vi "Linux Native Sleep Performance Test.vi"() -> ()   [LabVIEW 2021]
uses:
  <vilib>/Platform/TimedLoop/XDataNode/timing_clust.ctl
  <vilib>/Platform/TimedLoop/XDataNode/nitl_modes.ctl
  <vilib>/Platform/TimedLoop/XDataNode/wakeup.ctl
  <vilib>/NI/NI Linux RT Utilities/Controls/Public/nanosleep flags.ctl
  <vilib>/NI/NI Linux RT Utilities/Controls/Public/C Enums/clockid_t.ctl
  <vilib>/NI/NI Linux RT Utilities/VIs/Private/C Functions/clock_nanosleep.vi
  <vilib>/NI/NI Linux RT Utilities/VIs/Public/Convert Types/convert nanoseconds to timespec.vi
  <vilib>/NI/NI Linux RT Errno/VIs/Public/Generate LabVIEW Error from Errno.vi
  <vilib>/NI/NI Linux RT Errno/VIs/Public/Get Errno Value for Calling Thread.vi
  <vilib>/NI/NI Linux RT Errno/VIs/Public/Get LV Error Info from Errno.vi
  <vilib>/Utility/error.llb/Error Cluster From Error Code.vi
  <vilib>/Platform/TimedLoop/XDataNode/XDataNode.xnode
  <vilib>/Platform/TimedLoop/XDataNode/XDNodeRunTimeDep.lvlib
  <vilib>/NI/NI Linux RT Utilities/Linux RT Utilities.lvlib
panel:
  out "avg Linux Sleep":dbl
  out "max Linux Sleep":dbl
  out "avg RT Sleep":dbl
  out "max RT Sleep":dbl
  out "pass":bool
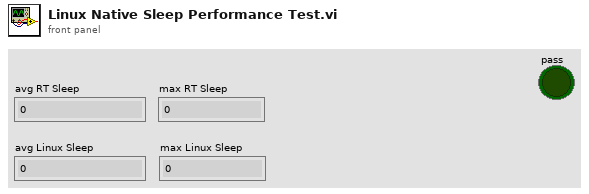
[diagram p1: front panel]
types:
  T1 = typedef "XDNodeRunTimeDep.lvlib/timing_clust.ctl" = cluster{"Expected End [f-1]":u64, "Actual End [f-1]":u64, "Finished Late? [f-1]":bool, "Expected End [i-1]":u64, "Actual End [i-1]":u64, "Finished Late? [i-1]":bool, "Expected Start [i]":u64, "Actual Start [i]":u64, "Expected Start [f]":u64, "Actual Start [f]":u64, "Source Name":string, "Structure Name":string, "Period":i64, "Deadline":i64, "Offset":i64, "Start":i64, "Priority":i32, "Timeout":i32, "Mode":T2, "Wakeup Reason":T3, "Error":errorcluster, "Source Type":string, "Secondary Source Type":string, "Global End Time":u64, "Global Start Time":u64, "Frame Duration":u64, "Iteration Duration":u64, "Assigned CPU":i32, "I/O Scan Engine Mode":u32}
  T2 = typedef "XDNodeRunTimeDep.lvlib/nitl_modes.ctl" = enum32{"No Change", "Process missed periods, maintain original phase", "Discard missed periods, maintain original phase", "Process missed periods, ignore original phase", "Discard missed periods, ignore original phase"}
  T3 = typedef "XDNodeRunTimeDep.lvlib/wakeup.ctl" = enum32{"Normal", "Aborted", "Asynchronous wakeup", "Timing source error", "Timed loop error", "Timeout"}
  T4 = typedef "Linux RT Utilities.lvlib/clockid_t.ctl" = enum16{"Realtime", "Monotonic"}
  T5 = typedef "Linux RT Utilities.lvlib/nanosleep flags.ctl" = enum16{"Relative Time", "Absolute Time"}
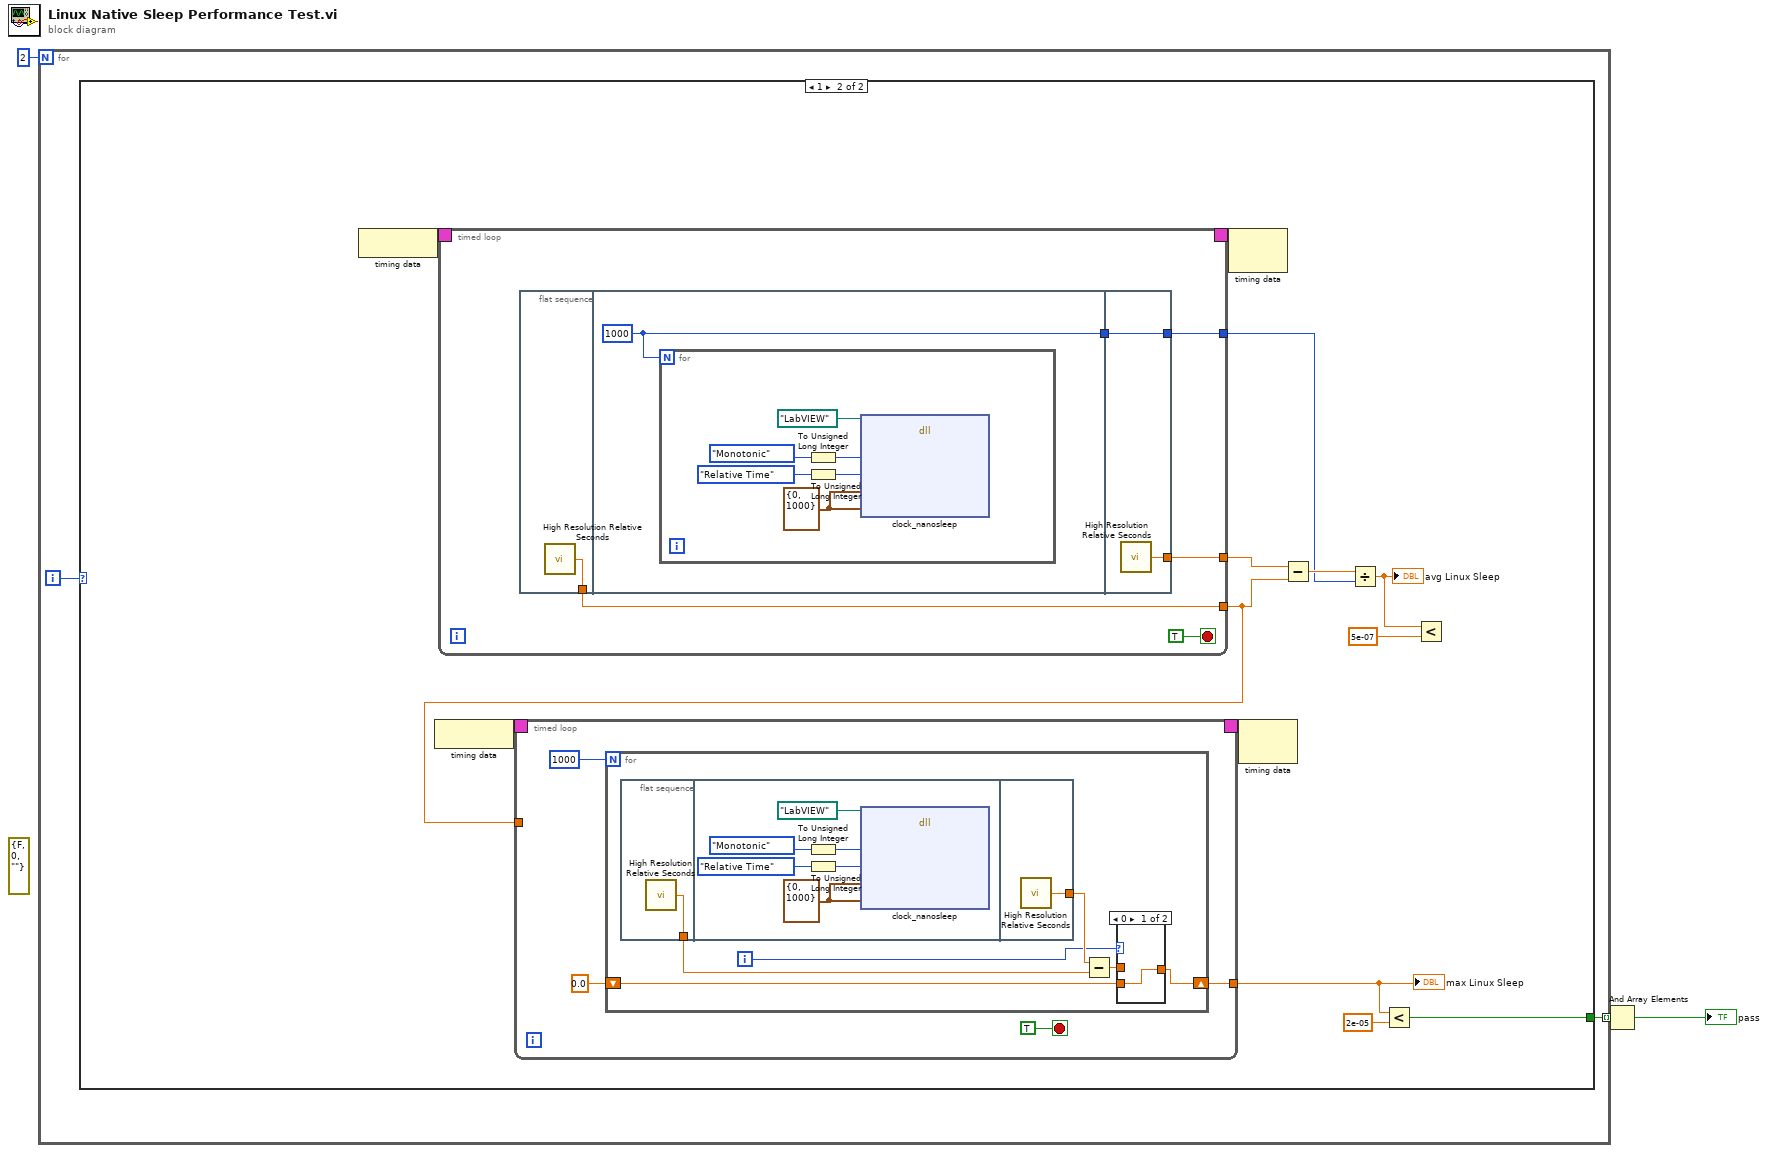
[diagram p0: block diagram]
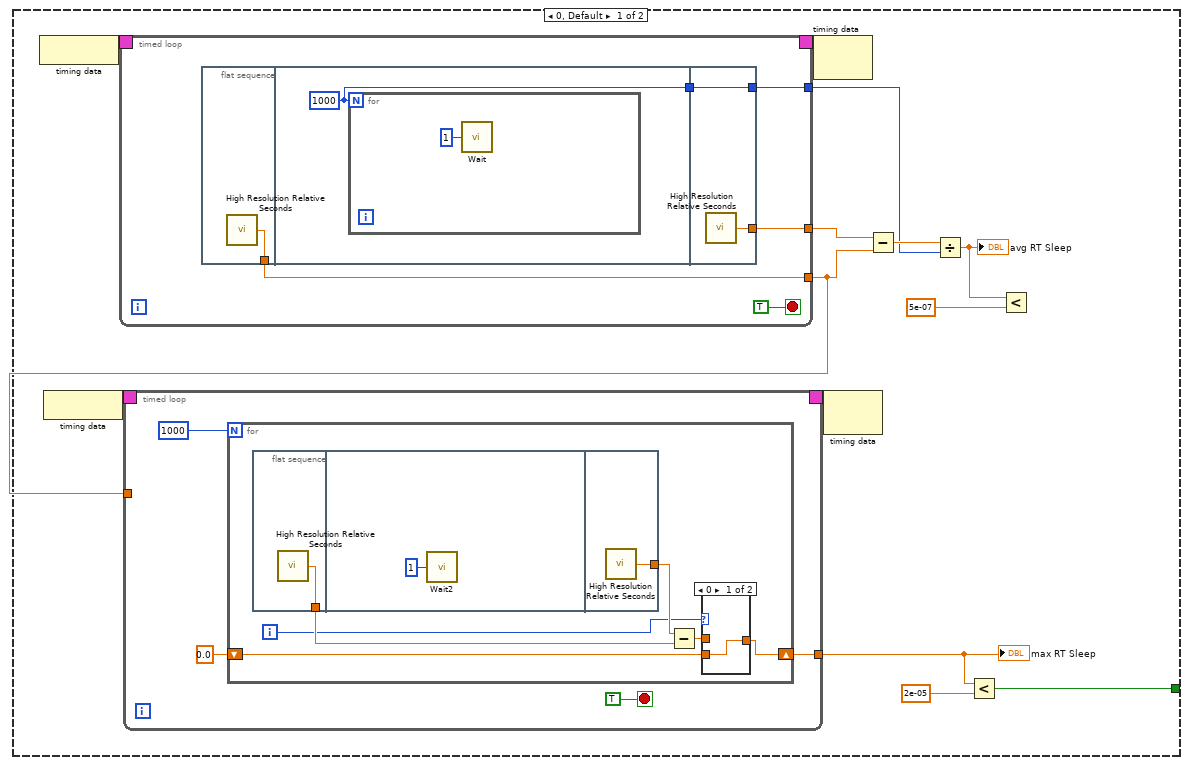
[diagram p2: hidden frame]
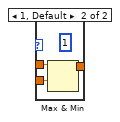
[diagram p3: hidden frame]
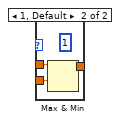
[diagram p4: hidden frame]
diagram:
  (unwired) errorcluster {"status"=FALSE, "code"=0, "source"=""} ("error out")
  n1 = for {
    N: 2 -> [_]
    tunnel: [w5] -> w2 mode=indexing
    i -> [w4]
    n2 = case shown="1" w4 {
      tunnel: [w7 w55] -> w5
      frame 0, Default {
        n3 = node-c288() -> (w18:T1)
        n4 = node-c288() -> (w16:T1)
        n5 = timed-loop {
          timing: w18 -> [_]
          timing-out: [_] -> w17
          tunnel: [w43] -> w14
          tunnel: [w42] -> w6
          tunnel: [w41] -> w12
          stop <- TRUE stop-if-true
          n6 = flat-sequence {
            tunnel: [w45] -> w42
            tunnel: [w46] -> w40
            tunnel: [w49] -> w43
            tunnel: [w48] -> w41
            tunnel: w40 -> [w48]
            frame #0 {
              n7 = call <vilib>:"High Resolution Relative Seconds.vi"() -> ("relative seconds"=w45:dbl)
            }
            frame #1 {
              w46 = 1000
              n8 = for {
                N: w46 -> [_]
                n9 = call "Wait"("Count(uSec)"=u32 1) -> ()  [unwired: 1 out]
              }
            }
            frame #2 {
              n10 = call <vilib>:"High Resolution Relative Seconds.vi"() -> ("relative seconds"=w49:dbl)
            }
          }
        }
        n11 = timed-loop {
          timing: w16 -> [_]
          timing-out: [_] -> w15
          tunnel: [w19] -> w9
          tunnel: w6 -> [_]
          stop <- TRUE stop-if-true
          n12 = for {
            N: 1000 -> [_]
            shift-right: [w24] -> w19
            shift-left: 0.0 -> [w25]
            i -> [w23]
            n13 = flat-sequence {
              tunnel: [w33] -> w27
              tunnel: [w35] -> w28
              frame #0 {
                n14 = call <vilib>:"High Resolution Relative Seconds.vi"() -> ("relative seconds"=w33:dbl)
              }
              frame #1 {
                n15 = call "Wait2"("Count(uSec)"=u32 1) -> ()  [unwired: 1 out]
              }
              frame #2 {
                n16 = call <vilib>:"High Resolution Relative Seconds.vi"() -> ("relative seconds"=w35:dbl)
              }
            }
            n17 = Subtract(x=w28, y=w27) -> (x-y=w26:dbl)
            n18 = case shown="0" w23 {
              tunnel: w26 -> [_ w32]
              tunnel: w25 -> [w29 w31]
              tunnel: [w29 w30] -> w24
              frame 0 {
              }
              frame 1, Default {
                (unwired) u32 1 ("milliseconds to wait")
                n19 = Max & Min(x=w32, y=w31) -> (max(x,y)=w30:dbl)  [unwired: 1 out]
              }
            }
          }
        }
        "max RT Sleep" <- w9
        n20 = node-c288(w17) -> ()  [unwired: 1 out]
        n21 = node-c288(w15) -> ()  [unwired: 1 out]
        n22 = Subtract(x=w14, y=w6) -> (x-y=w13:dbl)
        n23 = Divide(x=w13, y=w12) -> (x/y=w11:dbl)
        "avg RT Sleep" <- w11
        n24 = Less?(x=w9, y=2e-05) -> (x < y?=w7:bool)
        n25 = Less?(x=w11, y=5e-07) -> ()  [unwired: 1 out]
      }
      frame 1 {
        n26 = node-c288() -> (w66:T1)
        n27 = node-c288() -> (w64:T1)
        n28 = timed-loop {
          timing: w66 -> [_]
          timing-out: [_] -> w65
          tunnel: [w96] -> w62
          tunnel: [w95] -> w54
          tunnel: [w94] -> w60
          stop <- TRUE stop-if-true
          n29 = flat-sequence {
            tunnel: [w98] -> w95
            tunnel: [w99] -> w93
            tunnel: [w107] -> w96
            tunnel: [w106] -> w94
            tunnel: w93 -> [w106]
            frame #0 {
              n30 = call <vilib>:"High Resolution Relative Seconds.vi"() -> ("relative seconds"=w98:dbl)
            }
            frame #1 {
              w99 = 1000
              n31 = for {
                N: w99 -> [_]
                w100 = cluster{"sec":i64, "nsec":i64} {"sec"=0, "nsec"=1000} ("request")
                n32 = To Unsigned Long Integer(number=clockid_t."Monotonic" ("clockid_t")) -> (unsigned 32bit integer=w102:u32)
                n33 = To Unsigned Long Integer(number=nanosleep_flags."Relative Time" ("flags")) -> (unsigned 32bit integer=w101:u32)
                n34 = dll-call lib="?" fn="clock_nanosleep"(path in=path "LabVIEW" ("Path"), "clockid_t"=w102, "flags"=w101, "request"=w100, "remain"=w100) -> ()  [unwired: 7 in, 2 out]
              }
            }
            frame #2 {
              n35 = call <vilib>:"High Resolution Relative Seconds.vi"() -> ("relative seconds"=w107:dbl)
            }
          }
        }
        n36 = timed-loop {
          timing: w64 -> [_]
          timing-out: [_] -> w63
          tunnel: [w67] -> w57
          tunnel: w54 -> [_]
          stop <- TRUE stop-if-true
          n37 = for {
            N: 1000 -> [_]
            shift-right: [w72] -> w67
            shift-left: 0.0 -> [w73]
            i -> [w71]
            n38 = flat-sequence {
              tunnel: [w81] -> w75
              tunnel: [w88] -> w76
              frame #0 {
                n39 = call <vilib>:"High Resolution Relative Seconds.vi"() -> ("relative seconds"=w81:dbl)
              }
              frame #1 {
                w87 = cluster{"sec":i64, "nsec":i64} {"sec"=0, "nsec"=1000} ("request")
                n40 = To Unsigned Long Integer(number=clockid_t."Monotonic" ("clockid_t")) -> (unsigned 32bit integer=w85:u32)
                n41 = To Unsigned Long Integer(number=nanosleep_flags."Relative Time" ("flags")) -> (unsigned 32bit integer=w86:u32)
                n42 = dll-call lib="?" fn="clock_nanosleep"(path in=path "LabVIEW" ("Path"), "clockid_t"=w85, "flags"=w86, "request"=w87, "remain"=w87) -> ()  [unwired: 7 in, 2 out]
              }
              frame #2 {
                n43 = call <vilib>:"High Resolution Relative Seconds.vi"() -> ("relative seconds"=w88:dbl)
              }
            }
            n44 = Subtract(x=w76, y=w75) -> (x-y=w74:dbl)
            n45 = case shown="0" w71 {
              tunnel: w74 -> [_ w80]
              tunnel: w73 -> [w77 w79]
              tunnel: [w77 w78] -> w72
              frame 0 {
              }
              frame 1, Default {
                (unwired) u32 1 ("milliseconds to wait")
                n46 = Max & Min(x=w80, y=w79) -> (max(x,y)=w78:dbl)  [unwired: 1 out]
              }
            }
          }
        }
        "max Linux Sleep" <- w57
        n47 = node-c288(w65) -> ()  [unwired: 1 out]
        n48 = node-c288(w63) -> ()  [unwired: 1 out]
        n49 = Subtract(x=w62, y=w54) -> (x-y=w61:dbl)
        n50 = Divide(x=w61, y=w60) -> (x/y=w59:dbl)
        "avg Linux Sleep" <- w59
        n51 = Less?(x=w57, y=2e-05) -> (x < y?=w55:bool)
        n52 = Less?(x=w59, y=5e-07) -> ()  [unwired: 1 out]
      }
    }
  }
  n53 = And Array Elements(Boolean array=w2) -> (logical AND=→"pass":bool)
